vi "Configure Device.vi"(8 "error in (no error)":errorcluster, 10 "Max Beams":dbl, 11 "WS1041 in":refnum<class "WS1041.lvclass">) -> (0 "error out":errorcluster, 3 "WS1041 out":refnum<class "WS1041.lvclass">)   [LabVIEW 2020, in "WS1041.lvclass"]
uses:
  WS1041.lvclass
  Toggle 6.lvclass
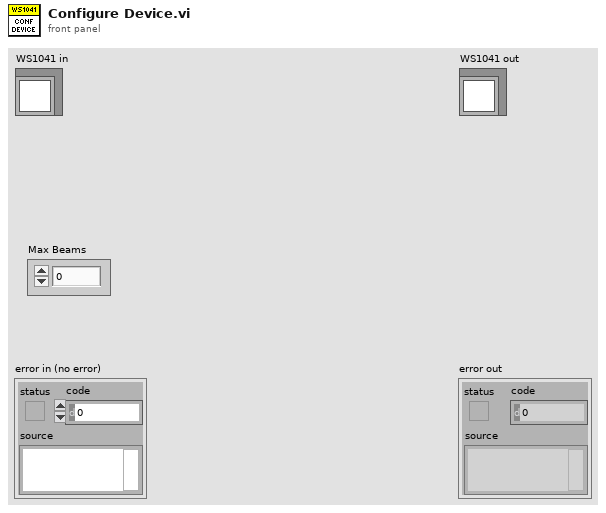
[diagram p1: front panel]
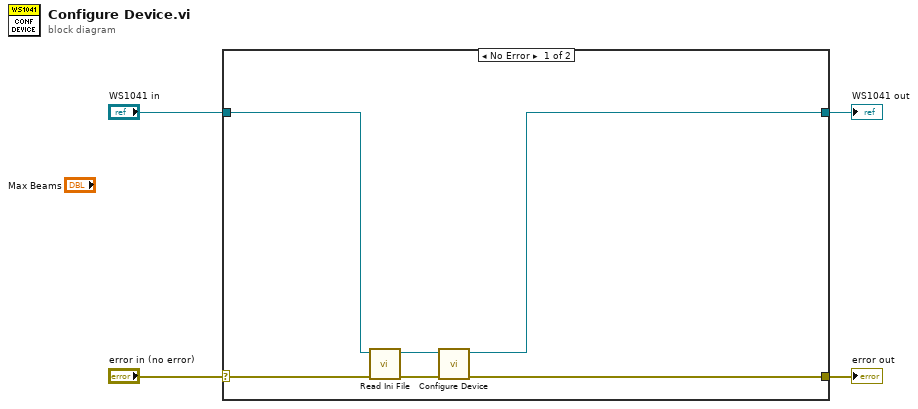
[diagram p0: block diagram]
diagram:
  n1 = case shown="No Error" "error in (no error)" {
    selector: "error in (no error)" -> [w10 w12]
    tunnel: [w7 w12] -> w3
    tunnel: [w5 w11] -> w1
    tunnel: "WS1041 in" -> [w9 w11]
    frame No Error {
      n2 = call "Read Ini File.vi"("error in (no error)"=w10, "WS1041 in"=w9) -> ("error out"=w8:errorcluster, "WS1041 out"=w6:refnum<class "WS1041.lvclass">)  [unwired: 8 in]
      n3 = call-parent "Configure Device.vi"("error in (no error)"=w8, "Toggle 6 in"=w6) -> ("error out"=w7:errorcluster, "Toggle 6 out"=w5:refnum<class "WS1041.lvclass">)  [unwired: 8 in]
    }
    frame Error {
    }
  }
  "error out" <- w3
  "WS1041 out" <- w1
